vi "Get Reception Data V.vi"(8 "error in (no error)":errorcluster, 11 "receptionStats":T1) -> (0 "error out":errorcluster, 2 "function return":i16, 3 "receptionStats out":T1)   [LabVIEW 2009, in "VantagePro.lvlib"]
doc: "DllAccess short int _stdcall GetStationFirmwareVersion_V ( char *verSt);DllAccess short int _stdcall GetReceptionData_V ( ReceptionStats *receptionStats);"
uses:
  VantagePro.lvlib
  <userlib>/VantagePro/VantagePro.dll
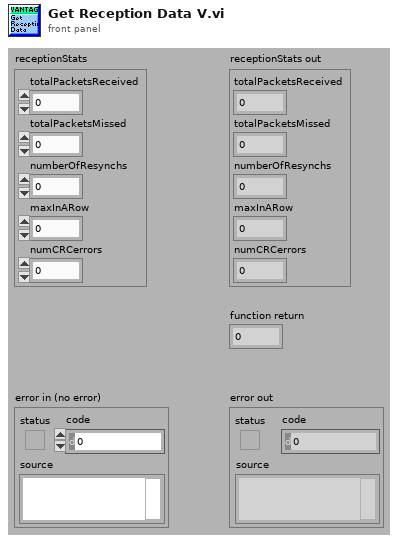
[diagram p1: front panel]
types:
  T1 = cluster{"totalPacketsReceived":i32, "totalPacketsMissed":i32, "numberOfResynchs":i32, "maxInARow":i32, "numCRCerrors":i32}
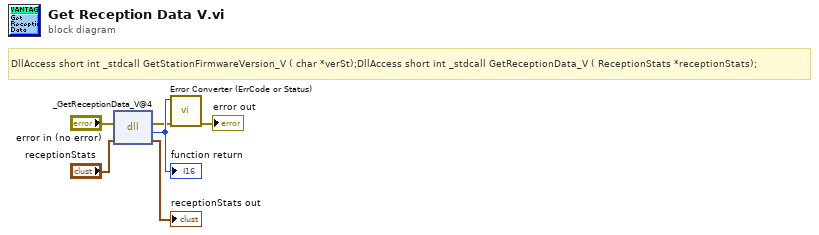
[diagram p0: block diagram]
diagram:
  # "DllAccess short int _stdcall GetStationFirmwareVersion_V ( char *verSt);DllAccess short int _stdcall GetReceptionData_V ( ReceptionStats *receptionStats);"
  n1 = dll-call lib="C:/Program Files/National Instruments/LabVIEW 2010/user.lib/VantagePro/VantagePro.*" fn="_GetReceptionData_V@4"(error in="error in (no error)", "receptionStats"="receptionStats") -> (error out=w2:errorcluster, w6:i16, "receptionStats"=→"receptionStats out":T1)  [unwired: 2 in, 1 out]
  "function return" <- w6
  n2 = call "Error Converter (ErrCode or Status).vi"("error in (no error)"=w2, "error code"=w6) -> ("error out"=→"error out":errorcluster)  [unwired: 9 in]
